vi "Tektronix DPO MSO 2000 4000 Series Acquire Waveform Measurement.vi"() -> ()   [LabVIEW 2009]
doc: "This example illustrates how to configure and read waveform measurement from the immediate measurement or specified displayed measurement using the following steps:\n\n1. Specify a valid VISA session. \n2. Configure measurement in reference level or in absolute level. \n3. Configure the measurement source and the corresponding parameters.\n4. Run the VI."
uses:
  <instrlib>/Tektronix DPO MSO 2000 4000 Series/Tektronix DPO MSO 2000 4000 Series.lvlib
panel:
  in  "Gating (0: Screen)":u16(ring) items=["Screen", "Between Cursors", "Off"]
  in  "Second Source Mid Ref":dbl=50.0
  in  "Ref Level Calculate Method (0: Auto Select)":i32(ring) items=["Auto Select", "Histogram", "Min/Max"]
  in  "Low Ref":dbl=10.0
  in  "Mid Ref":dbl=50.0
  in  "High Ref":dbl=90.0
  in  "Level Type (0: Reference Level)":u16(ring) items=["Reference Level", "Absolute Level"]
  out "Measurement Value":dbl
  in  "Measurement Number (0: Measurement 1)":i32(ring) items=["Measurement 1", "Measurement 2", "Measurement 3", "Measurement 4"]
  in  "Destination Channel (1: Channel 2)":u16(ring)=1 items=["Channel 1", "Channel 2", "Channel 3", "Channel 4", "Math", "D0", "D1", "D2", "D3", "D4", "D5", "D6", "D7", "D8", "D9", "D10", "D11", "D12", "D13", "D14", "D15", "Reference 1", "Reference 2", "Reference 3", "Reference 4", "Amplitude", "Frequency", "Phase"]
  in  "Measurement Function (21: Period)":i32(ring)=21 items=["Amplitude", "Area", "Burst Width", "Cycle Area", "Voltage Mean (cycle)", "Voltage RMS (cycle)", "Delay", "Fall Time", "Frequency", "Voltage High", "Voltage Low", "Voltage Max", "Voltage Mean", "Voltage Min", "Negative Duty Cycle", "Negative Edges Count", "Negative Overshoot", "Negative Pulses Count", "Negative Pulse Width", "Positive Duty Cycle", "Positive Edges Count", "Period", "Phase", "Vpp", "Positive Overshoot", "Positive Pulses Count", "Positive Pulse Width", "Rise Time", "Voltage RMS"]
  in  "Maximum Time (10000 ms)":u32=10000
  in  "Channel (0: Channel 1)":u16(ring) items=["Channel 1", "Channel 2", "Channel 3", "Channel 4", "Math", "D0", "D1", "D2", "D3", "D4", "D5", "D6", "D7", "D8", "D9", "D10", "D11", "D12", "D13", "D14", "D15", "Reference 1", "Reference 2", "Reference 3", "Reference 4", "Amplitude", "Frequency", "Phase"]
  in  "Measurement Source (0: Immediate)":u16(ring) items=["Immediate", "Memory"]
  in  "VISA resource name":refnum<visa-resource-name>
  # "(C) 2006 - 2013. National Instruments Corporation. ALL RIGHTS RESERVED."
  # "Configures Measurement in reference level or in absolute level according to Level Type control.\n\nNotes:\n\nThe unit of the following control is Volts in absolute level, and the values shold be changed to a meaningful values:\nHigh Ref\nMid Ref\nLow Ref\nSecond Source Mid Ref"
  # "Since the instrument contains four displayed measurements and one immediate measurement, You can obtain measurement results by using Read Waveform Measurement VI from the immediate measurement or Read Waveform Measurement In Memory VI from the specified displayed measurement, which is decided by Measurement Type control."
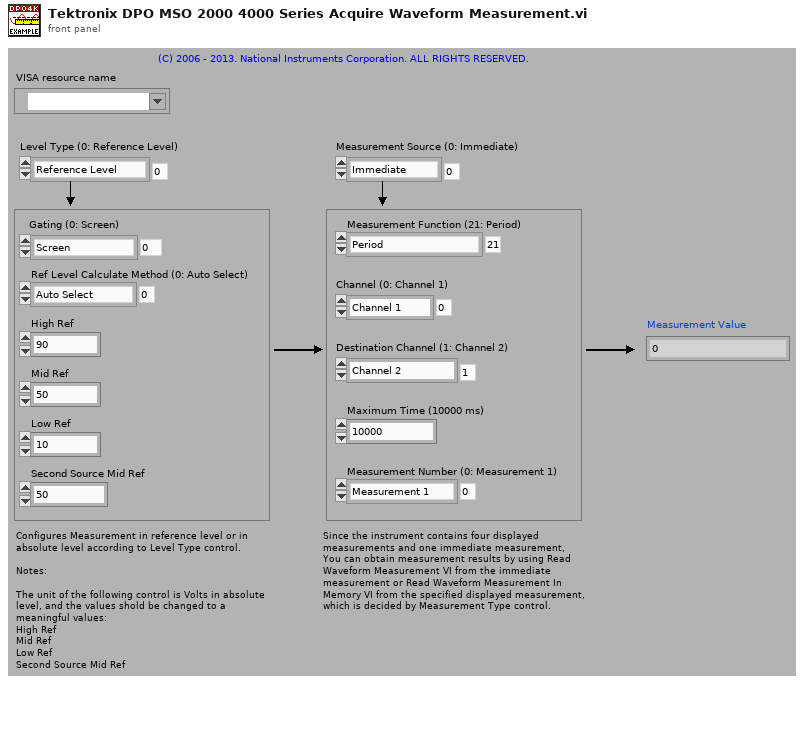
[diagram p1: front panel]
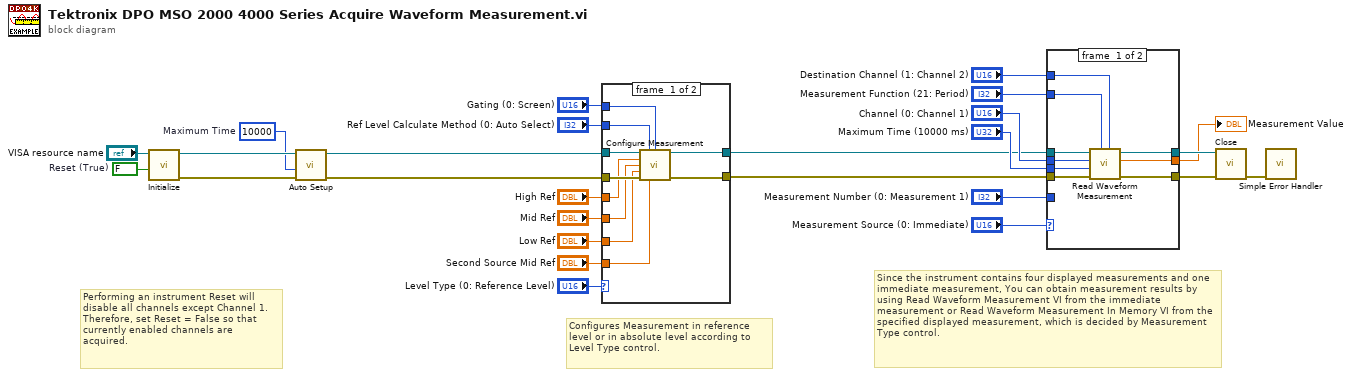
[diagram p0: block diagram]
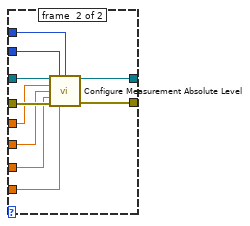
[diagram p2: hidden frame]
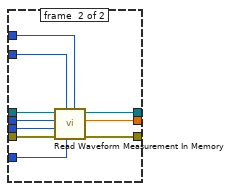
[diagram p3: hidden frame]
diagram:
  w1 = 10000  # Maximum Time
  w15 = FALSE  # Reset (True)
  # "Since the instrument contains four displayed measurements and one immediate measurement, You can obtain measurement results by using Read Waveform Measurement VI from the immediate measurement or Read Waveform Measurement In Memory VI from the specified displayed measurement, which is decided by Measurement Type control."
  # "Configures Measurement in reference level or in absolute level according to Level Type control."
  # "Performing an instrument Reset will disable all channels except Channel 1. Therefore, set Reset = False so that currently enabled channels are acquired."
  n1 = call <instrlib>:"Initialize.vi"("Reset (True)"=w15, "VISA resource name"="VISA resource name") -> ("error out"=w2:errorcluster, "VISA resource name out"=w3:refnum<visa-resource-name>)  [unwired: 8 in]
  n2 = call <instrlib>:"Auto Setup.vi"("error in (no error)"=w2, "Maximum Time (10000ms)"=w1, "VISA resource name"=w3) -> ("error out"=w4:errorcluster, "VISA resource name out"=w5:refnum<visa-resource-name>)  [unwired: 7 in]
  n3 = case shown="0, Default" "Level Type (0: Reference Level)" {
    tunnel: w5 -> [w36 w46]
    tunnel: w4 -> [w35 w45]
    tunnel: [w33 w44] -> w7
    tunnel: [w34 w43] -> w6
    tunnel: "Gating (0: Screen)" -> [w32 w37]
    tunnel: "Ref Level Calculate Method (0: Auto Select)" -> [w31 w39]
    tunnel: "High Ref" -> [w30 w40]
    tunnel: "Mid Ref" -> [w29 w41]
    tunnel: "Low Ref" -> [w28 w42]
    tunnel: "Second Source Mid Ref" -> [w27 w38]
    frame #0 {
      n4 = call <instrlib>:"Configure Measurement.vi"("VISA resource name"=w36, "Ref Level Calculate Method (0: Auto Select)"=w31, "Gating (0: Screen)"=w32, "High Ref (90%)"=w30, "Mid Ref (50%)"=w29, "Low Ref (10%)"=w28, "error in (no error)"=w35, "Second Source Mid Ref (50%)"=w27) -> ("VISA resource name out"=w33:refnum<visa-resource-name>, "error out"=w34:errorcluster)  [unwired: 6 in]
    }
    frame #1 {
      n5 = call <instrlib>:"Configure Measurement Absolute Level.vi"("VISA resource name"=w46, "Ref Level Calculate Method (0: Auto Select)"=w39, "Gating (0: Screen)"=w37, "High Ref (0 V)"=w40, "Mid Ref (0 V)"=w41, "Low Ref (0 V)"=w42, "error in (no error)"=w45, "Second Source Mid Ref (0 V)"=w38) -> ("VISA resource name out"=w44:refnum<visa-resource-name>, "error out"=w43:errorcluster)  [unwired: 6 in]
    }
  }
  n6 = case shown="0, Default" "Measurement Source (0: Immediate)" {
    tunnel: [w51 w65] -> w23
    tunnel: [w50 w64] -> w22
    tunnel: "Channel (0: Channel 1)" -> [w55 w63]
    tunnel: "Maximum Time (10000 ms)" -> [w54 w62]
    tunnel: "Measurement Function (21: Period)" -> [w53 w61]
    tunnel: "Destination Channel (1: Channel 2)" -> [w52 w60]
    tunnel: "Measurement Number (0: Measurement 1)" -> [_ w59]
    tunnel: [w49 w58] -> w17
    tunnel: w7 -> [w47 w57]
    tunnel: w6 -> [w48 w56]
    frame #0 {
      n7 = call <instrlib>:"Read Waveform Measurement.vi"("Destination Channel (1: Channel 2)"=w52, "Measurement Function (0: Period)"=w53, "error in (no error)"=w48, "Maximum Time (10000ms)"=w54, "Channel (0: Channel 1)"=w55, "VISA resource name"=w47) -> ("error out"=w50:errorcluster, "Measurement Value"=w49:dbl, "VISA resource name out"=w51:refnum<visa-resource-name>)  [unwired: 3 in]
    }
    frame #1 {
      n8 = call <instrlib>:"Read Waveform Measurement In Memory.vi"("Destination Channel (1: Channel 2)"=w60, "Measurement Number (0: Measurement 1)"=w59, "Measurement Function (21: Period)"=w61, "error in (no error)"=w56, "Maximum Time (10000 ms)"=w62, "Channel (0: Channel 1)"=w63, "VISA resource name"=w57) -> ("error out"=w64:errorcluster, "Measurement Value"=w58:dbl, "VISA resource name out"=w65:refnum<visa-resource-name>)  [unwired: 2 in]
    }
  }
  "Measurement Value" <- w17
  n9 = call <instrlib>:"Close.vi"("error in (no error)"=w22, "VISA resource name"=w23) -> ("error out"=w24:errorcluster)  [unwired: 9 in]
  n10 = call <vilib>:"Simple Error Handler.vi"("error in (no error)"=w24) -> ()  [unwired: 4 in, 5 out]
